vi "Ramp_Trajectory_v2.vi"(7 "Initial Time (s)":dbl, 8 "Period (s)":dbl, 9 "Ramp Duration (s)":dbl, 10 "Final Position (deg)":dbl, 11 "Initial Position (deg)":dbl) -> (3 "Profile 2":cluster{"time (s)":dbl, "setpoint":dbl}[](array[cluster]) {"setpoint" format="%.2f"; "time (s)" format="%.3f"})   [LabVIEW 2019]
uses:
  <vilib>/Analysis/1siggen.llb/Ramp Pattern by Samples.vi
  <vilib>/Analysis/NI_AALBase.lvlib
panel:
  out "XY Graph":cluster{"X":dbl, "Y":dbl}[](graph)
  out "Waveform Graph":waveform(dbl)(graph)
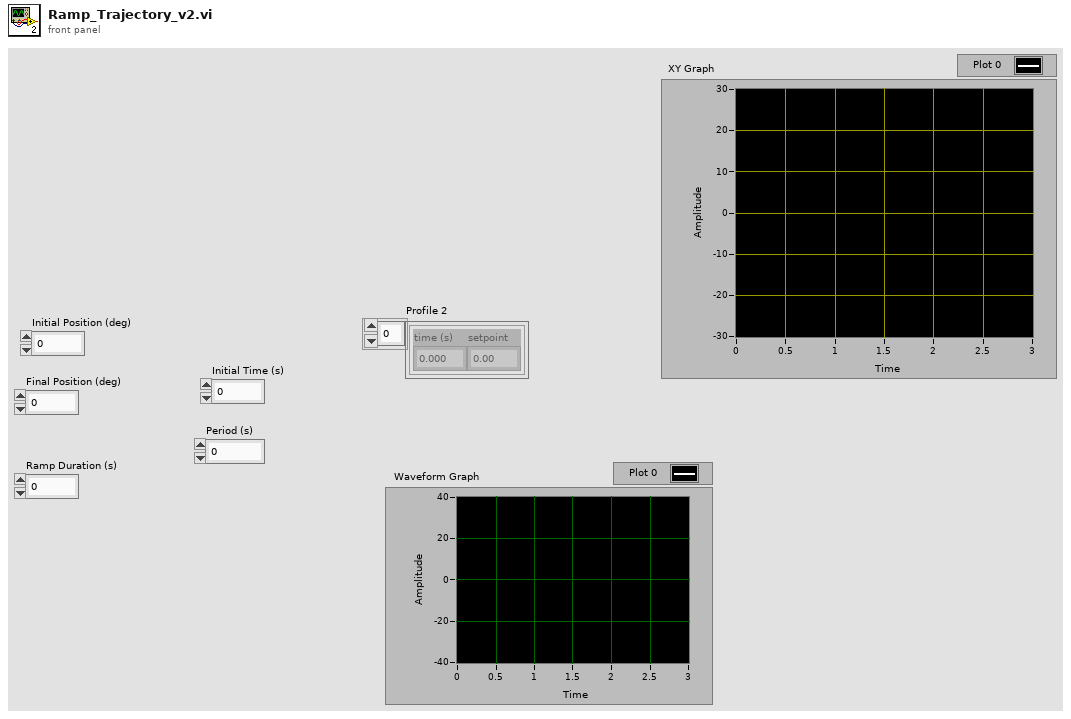
[diagram p1: front panel]
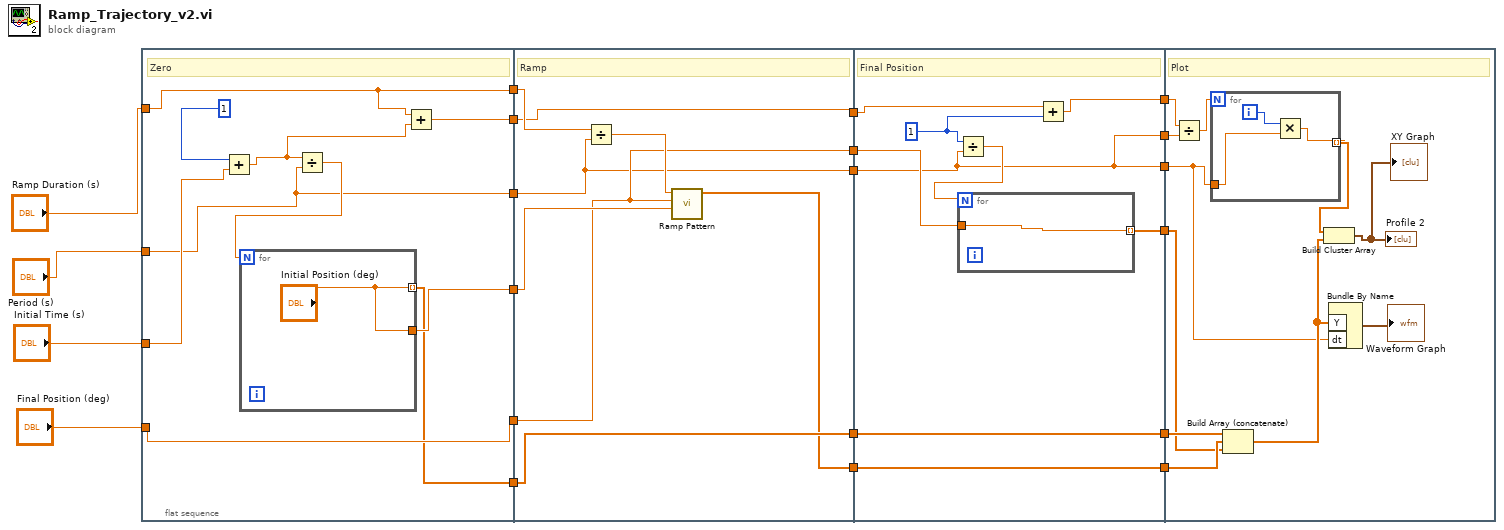
[diagram p0: block diagram]
diagram:
  n1 = flat-sequence {
    tunnel: "Initial Time (s)" -> [w30]
    tunnel: "Period (s)" -> [w26]
    tunnel: "Ramp Duration (s)" -> [w23]
    tunnel: [w23] -> w18
    tunnel: [w28] -> w17
    tunnel: [w27] -> w16
    tunnel: "Final Position (deg)" -> [w27]
    tunnel: [w26] -> w14
    tunnel: [w25] -> w13
    tunnel: [w22] -> w7
    tunnel: w18 -> [w35]
    tunnel: w17 -> [w40]
    tunnel: w16 -> [w36]
    tunnel: w14 -> [w34]
    tunnel: w13 -> [w38]
    tunnel: [w38] -> w11
    tunnel: [w37] -> w9
    tunnel: [w36] -> w8
    tunnel: w7 -> [w33]
    tunnel: [w34] -> w6
    tunnel: [w33] -> w3
    tunnel: [w49] -> w12
    tunnel: w11 -> [w49]
    tunnel: [w42] -> w10
    tunnel: w9 -> [w42]
    tunnel: w8 -> [w48]
    tunnel: w6 -> [w41]
    tunnel: [w47] -> w5
    tunnel: [w41] -> w4
    tunnel: w3 -> [w45]
    tunnel: [w43] -> w2
    tunnel: [w41] -> w1
    tunnel: w12 -> [w61]
    tunnel: w10 -> [w60]
    tunnel: w5 -> [w59]
    tunnel: w4 -> [w55]
    tunnel: w2 -> [w54]
    tunnel: w1 -> [w52]
    frame #0 {
      # "Zero"
      n2 = Add(x=1, y=w30) -> (x+y=w24:dbl)
      n3 = Divide(x=w24, y=w26) -> (x/y=w29:dbl)
      n4 = for {
        N: w29 -> [_]
        tunnel: ["Initial Position (deg)"] -> w25 mode=indexing
        tunnel: ["Initial Position (deg)"] -> w28
      }
      n5 = Add(x=w23, y=w24) -> (x+y=w22:dbl)
    }
    frame #1 {
      # "Ramp"
      n6 = Divide(x=w35, y=w34) -> (x/y=w39:dbl)
      n7 = call-poly <vilib>:"Ramp Pattern.vi"("start"=w40, "end"=w36, "samples"=w39) -> ("Ramp Pattern"=w37:dbl[])  [unwired: 7 in, 1 out]
    }
    frame #2 {
      w44 = 1
      # "Final Position"
      n8 = Divide(x=w44, y=w41) -> (x/y=w46:dbl)
      n9 = for {
        N: w46 -> [_]
        tunnel: [w50] -> w47 mode=indexing
        tunnel: w48 -> [w50]
      }
      n10 = Add(x=w45, y=w44) -> (x+y=w43:dbl)
    }
    frame #3 {
      # "Plot"
      n11 = Divide(x=w54, y=w52) -> (x/y=w53:dbl)
      n12 = for {
        N: w53 -> [_]
        tunnel: w55 -> [w63]
        tunnel: [w62] -> w58 mode=indexing
        i -> [w64]
        n13 = Multiply(x=w64, y=w63) -> (x*y=w62:dbl)
      }
      n14 = Build Array (concatenate)(w61, w60, w59) -> (w56:dbl[])
      n15 = Build Cluster Array(w58, w56) -> (→"Profile 2" →"XY Graph":cluster{dbl, "Final Position (deg) ":dbl}[])
      n16 = Bundle By Name("Y"=w56, "dt"=w55) -> (→"Waveform Graph":waveform(dbl))  [unwired: 1 in]
    }
  }
